vi "getBorderNum.vi"(0 "Refnum in":T1, 2 "Cut Limit":dbl format="%#_13g", 5 "Bounding Box":cluster{"x":sgl, "y":sgl}[][](array[cluster]), 7 "Position":sgl[][](array[numeric]), 9 "Angle":sgl[](array[numeric]), 11 "error in (no error)":errorcluster, 12 "Step":sgl=0.29742944, 13 "Origin Pixel":dbl[](array[numeric])) -> (4 "Refnum out":T1, 8 "Data Pieces":T3(array[cluster]) {"ROI Números"."Contours"."Type" items=["No Selection", "Point", "Line", "Rectangle", "Oval", "Polygon", "Freehand Region", "Annulus", "Unused2", "Unused3", "Broken Line", "Freehand Line", "Rotated Rectangle"]}, 15 "error out":errorcluster)   [LabVIEW 2016]
uses:
  <vilib>/vision/Image Controls.llb/IMAQ Image.ctl
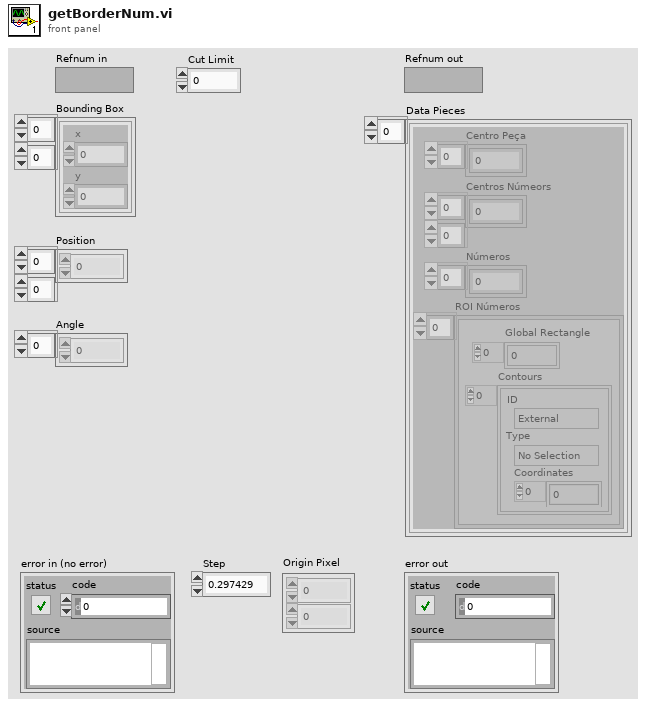
[diagram p1: front panel]
types:
  T1 = typedef "IMAQ Image.ctl" = refnum<image>
  T2 = typedef "ROI Descriptor" = cluster{"Global Rectangle":i32[], "Contours":cluster{"ID":enum32{"External", "Internal"}, "Type":u32, "Coordinates":i32[]}[]}
  T3 = cluster{"Centro Peça":dbl[], "Centros Númeors":dbl[][], "Números":u8[], "ROI Números":T2[]}[]
  T4 = cluster{"Centro Peça":dbl[], "Centros Númeors":dbl[][], "Números":u8[], "ROI Números":T2[]}
  T5 = typedef "IMAQ Rectangle" = cluster{"Left":i32, "Top":i32, "Right":i32, "Bottom":i32, "Rotation":dbl}
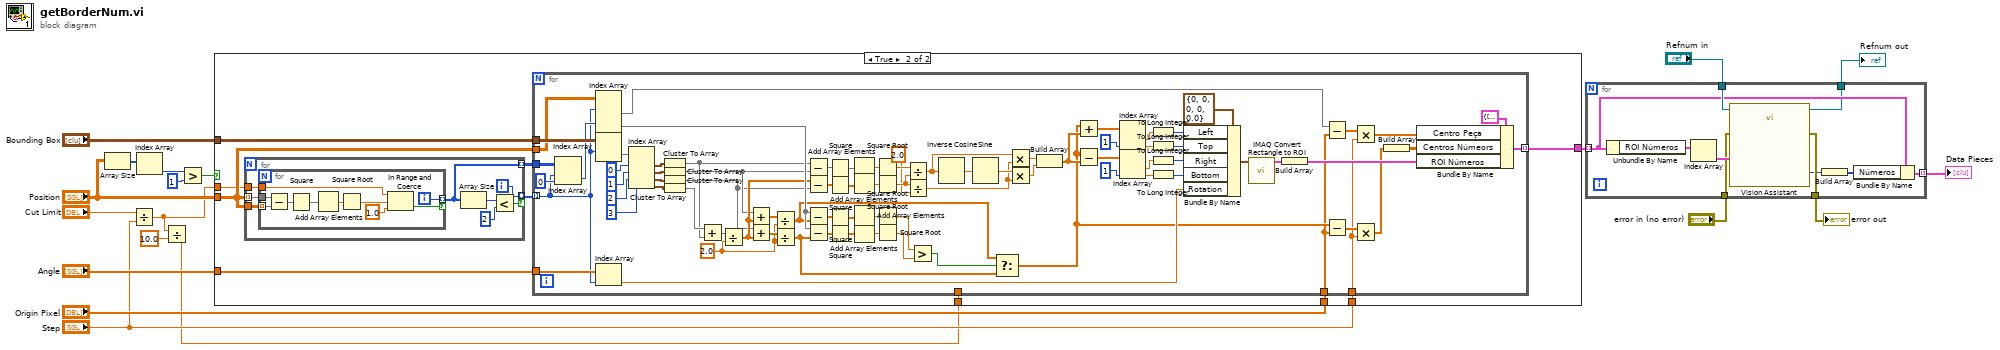
[diagram p0: block diagram]
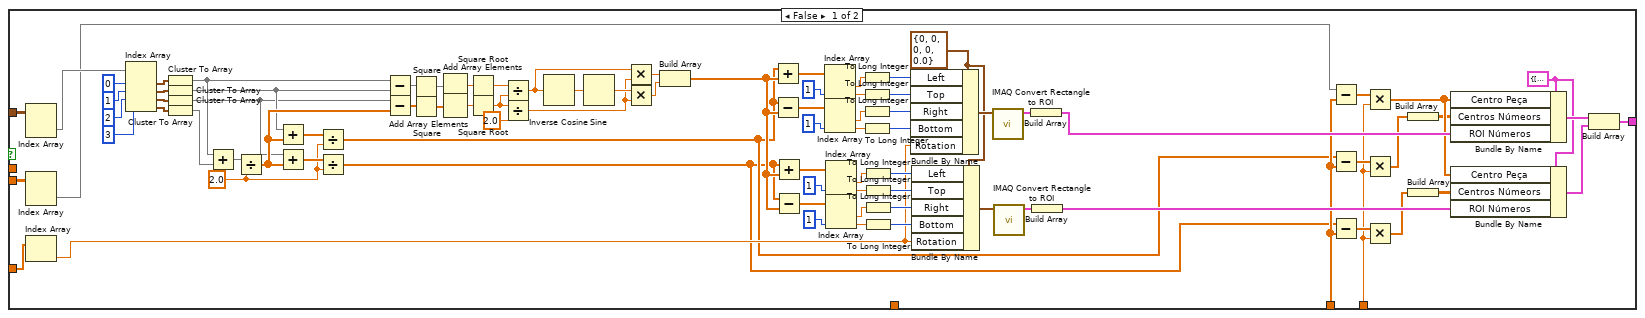
[diagram p2: hidden frame]
diagram:
  n1 = Array Size(array="Position") -> (size(s)=w9:i32[])
  n2 = Divide(x="Cut Limit", y="Step") -> (x/y=w3:dbl)
  n3 = Index Array(array=w9) -> (element=w10:i32)  [unwired: 1 in]
  n4 = Divide(x=w3, y=10.0) -> (x/y=w1:dbl)
  n5 = Greater?(x=w10, y=1) -> (0:w8:bool)
  n6 = case shown="True" w8 {
    tunnel: "Bounding Box" -> [w105 w115]
    tunnel: "Position" -> [w104 w114]
    tunnel: "Angle" -> [w43 w112]
    tunnel: [w39 w110] -> w14
    tunnel: w3 -> [_ w109]
    tunnel: "Origin Pixel" -> [w26 w108]
    tunnel: "Step" -> [w27 w107]
    tunnel: w1 -> [_ w106]
    frame False {
      w38 = T4 {"Centro Peça"=[0.0, 0.0], "Centros Númeors"=[[0.0, 0.0], [0.0, 0.0]], "Números"=[0, 0], "ROI Números"=[]} ("Dados Peça")
      w44 = T5 {"Left"=0, "Top"=0, "Right"=0, "Bottom"=0, "Rotation"=0.0} ("Rectangle")
      w80 = 2.0 ("y")
      n7 = Index Array(array=w105) -> (element=w103:cluster{"x":sgl, "y":sgl}[])  [unwired: 2 in]
      n8 = Index Array(array=w104) -> (element=w31:sgl[])  [unwired: 2 in]
      n9 = Index Array(array=w43) -> (element=w42:sgl)  [unwired: 1 in]
      n10 = Index Array(array=w103, index #1=0 ("index"), index #2=1 ("index"), index #3=2 ("index"), index #4=3 ("index")) -> (element #1=w98:cluster{"x":sgl, "y":sgl}, element #2=w97:cluster{"x":sgl, "y":sgl}, element #3=w96:cluster{"x":sgl, "y":sgl}, element #4=w95:cluster{"x":sgl, "y":sgl})
      n11 = Cluster To Array(cluster=w98) -> (array=w86:sgl[])
      n12 = Cluster To Array(cluster=w97) -> (array=w84:sgl[])
      n13 = Cluster To Array(cluster=w96) -> (array=w83:sgl[])
      n14 = Cluster To Array(cluster=w95) -> (array=w91:sgl[])
      n15 = Add(x=w86, y=w91) -> (x+y=w90:sgl[])
      n16 = Divide(x=w90, y=w80) -> (x/y=w85:dbl[])
      n17 = Add(x=w84, y=w85) -> (x+y=w82:dbl[])
      n18 = Add(x=w83, y=w85) -> (x+y=w81:dbl[])
      n19 = Divide(x=w82, y=w80) -> (x/y=w25:dbl[])
      n20 = Divide(x=w81, y=w80) -> (x/y=w24:dbl[])
      n21 = Subtract(x=w86, y=w84) -> (x-y=w87:sgl[])
      n22 = Subtract(x=w83, y=w85) -> (x-y=w92:dbl[])
      n23 = Square(x=w87) -> (x^2=w89:sgl[])
      n24 = Square(x=w92) -> (x^2=w94:dbl[])
      n25 = Add Array Elements(numeric array=w89) -> (sum=w88:sgl)
      n26 = Add Array Elements(numeric array=w94) -> (sum=w93:dbl)
      n27 = Square Root(x=w88) -> (sqrt(x)=w79:sgl)
      n28 = Square Root(x=w93) -> (sqrt(x)=w78:dbl)
      n29 = Divide(x=w79, y=w78) -> (x/y=w72:dbl)
      n30 = Divide(x=w78, y=2.0) -> (x/y=w71:dbl)
      n31 = Inverse Cosine(1:w72) -> (0:w76:dbl)
      n32 = Sine(x=w76) -> (sin(x)=w75:dbl)
      n33 = Multiply(x=w72, y=w71) -> (x*y=w73:dbl)
      n34 = Multiply(x=w75, y=w71) -> (x*y=w74:dbl)
      n35 = Build Array(w73, w74) -> (w41:dbl[])
      n36 = Add(x=w25, y=w41) -> (x+y=w58:dbl[])
      n37 = Subtract(x=w25, y=w41) -> (x-y=w59:dbl[])
      n38 = Add(x=w24, y=w41) -> (x+y=w45:dbl[])
      n39 = Subtract(x=w24, y=w41) -> (x-y=w46:dbl[])
      n40 = Index Array(array=w58, index #2=1 ("index")) -> (element #1=w60:dbl, element #2=w61:dbl)  [unwired: 1 in]
      n41 = Index Array(array=w59, index #2=1 ("index")) -> (element #1=w62:dbl, element #2=w63:dbl)  [unwired: 1 in]
      n42 = Index Array(array=w45, index #2=1 ("index")) -> (element #1=w47:dbl, element #2=w48:dbl)  [unwired: 1 in]
      n43 = Index Array(array=w46, index #2=1 ("index")) -> (element #1=w49:dbl, element #2=w50:dbl)  [unwired: 1 in]
      n44 = To Long Integer(number=w60) -> (32bit integer=w67:i32)
      n45 = To Long Integer(number=w61) -> (32bit integer=w66:i32)
      n46 = To Long Integer(number=w62) -> (32bit integer=w65:i32)
      n47 = To Long Integer(number=w63) -> (32bit integer=w64:i32)
      n48 = To Long Integer(number=w47) -> (32bit integer=w54:i32)
      n49 = To Long Integer(number=w48) -> (32bit integer=w53:i32)
      n50 = To Long Integer(number=w49) -> (32bit integer=w52:i32)
      n51 = To Long Integer(number=w50) -> (32bit integer=w51:i32)
      n52 = Bundle By Name(cluster=w44, "Left"=w67, "Top"=w66, "Right"=w65, "Bottom"=w64, "Rotation"=w42) -> (w68:T5)
      n53 = Bundle By Name(cluster=w44, "Left"=w54, "Top"=w53, "Right"=w52, "Bottom"=w51, "Rotation"=w42) -> (w55:T5)
      n54 = call "IMAQ Convert Rectangle to ROI"("Rectangle"=w68) -> ("ROI Descriptor"=w37:T2)  [unwired: 8 in, 1 out]
      n55 = call "IMAQ Convert Rectangle to ROI"("Rectangle"=w55) -> ("ROI Descriptor"=w36:T2)  [unwired: 8 in, 1 out]
      n56 = Build Array(w37) -> (w34:T2[])
      n57 = Build Array(w36) -> (w35:T2[])
      n58 = Subtract(x=w31, y=w26) -> (x-y=w32:dbl[])
      n59 = Subtract(x=w25, y=w26) -> (x-y=w29:dbl[])
      n60 = Subtract(x=w24, y=w26) -> (x-y=w28:dbl[])
      n61 = Multiply(x=w32, y=w27) -> (x*y=w30:dbl[])
      n62 = Multiply(x=w29, y=w27) -> (x*y=w23:dbl[])
      n63 = Multiply(x=w28, y=w27) -> (x*y=w20:dbl[])
      n64 = Build Array(w23) -> (w22:dbl[][])
      n65 = Build Array(w20) -> (w21:dbl[][])
      n66 = Bundle By Name(cluster=w38, "Centro Peça"=w30, "Centros Númeors"=w22, "ROI Números"=w34) -> (w40:T4)
      n67 = Bundle By Name(cluster=w38, "Centro Peça"=w30, "Centros Númeors"=w21, "ROI Números"=w35) -> (w33:T4)
      n68 = Build Array(w40, w33) -> (w39:T3)
    }
    frame True {
      n69 = for {
        tunnel: w114 -> [w204] mode=indexing
        tunnel: w114 -> [w203]
        tunnel: [w202] -> w113 mode=indexing if=w199
        tunnel: [w198] -> w111 mode=indexing
        tunnel: w109 -> [w197]
        i -> [w202]
        n70 = for {
          tunnel: w204 -> [w214]
          tunnel: w203 -> [w210] mode=indexing
          tunnel: [w207] -> w198 mode=indexing if=w206
          tunnel: w197 -> [w205]
          i -> [w207]
          n71 = Subtract(x=w214, y=w210) -> (x-y=w213:sgl[])
          n72 = Square(x=w213) -> (x^2=w212:sgl[])
          n73 = Add Array Elements(numeric array=w212) -> (sum=w211:sgl)
          n74 = Square Root(x=w211) -> (sqrt(x)=w208:sgl)
          n75 = In Range and Coerce(upper limit=w205, x=w208, lower limit=1.0) -> (In Range?=w206:bool)  [unwired: 1 out]
        }
        n76 = Array Size(array=w198) -> (size(s)=w201:i32)
        n77 = Less?(x=w201, y=2) -> (x < y?=w199:bool)
      }
      n78 = for {
        tunnel: w115 -> [w196]
        tunnel: w114 -> [w194]
        tunnel: w113 -> [w156] mode=indexing
        tunnel: w112 -> [w182]
        tunnel: w111 -> [w179]
        tunnel: [w128] -> w110 mode=indexing
        tunnel: w108 -> [w120]
        tunnel: w107 -> [w119]
        tunnel: w106 -> [_]
        w155 = 2.0 ("y")
        n79 = Index Array(array=w179, index (row)=w156, index (col)=0 ("disabled index (col)")) -> (element=w178:i32)
        n80 = Index Array(array=w194, index (row) #1=w156, index (row) #2=w178) -> (element #1=w127:sgl[], element #2=w157:sgl[])  [unwired: 2 in]
        n81 = Index Array(array=w196, index (row)=w156) -> (element=w195:cluster{"x":sgl, "y":sgl}[])  [unwired: 1 in]
        n82 = Index Array(array=w182, index=w156) -> (element=w181:sgl)
        n83 = Index Array(array=w195, index #1=0 ("index"), index #2=1 ("index"), index #3=2 ("index"), index #4=3 ("index")) -> (element #1=w192:cluster{"x":sgl, "y":sgl}, element #2=w193:cluster{"x":sgl, "y":sgl}, element #3=w191:cluster{"x":sgl, "y":sgl}, element #4=w174:cluster{"x":sgl, "y":sgl})
        n84 = Cluster To Array(cluster=w192) -> (array=w144:sgl[])
        n85 = Cluster To Array(cluster=w193) -> (array=w143:sgl[])
        n86 = Cluster To Array(cluster=w191) -> (array=w138:sgl[])
        n87 = Cluster To Array(cluster=w174) -> (array=w171:sgl[])
        n88 = Add(x=w171, y=w144) -> (x+y=w173:sgl[])
        n89 = Divide(x=w173, y=w155) -> (x/y=w149:dbl[])
        n90 = Add(x=w143, y=w149) -> (x+y=w148:dbl[])
        n91 = Add(x=w138, y=w149) -> (x+y=w170:dbl[])
        n92 = Divide(x=w148, y=w155) -> (x/y=w154:dbl[])
        n93 = Divide(x=w170, y=w155) -> (x/y=w153:dbl[])
        n94 = Subtract(x=w144, y=w143) -> (x-y=w145:sgl[])
        n95 = Subtract(x=w149, y=w138) -> (x-y=w152:dbl[])
        n96 = Subtract(x=w157, y=w154) -> (x-y=w169:dbl[])
        n97 = Subtract(x=w157, y=w153) -> (x-y=w158:dbl[])
        n98 = Square(x=w145) -> (x^2=w147:sgl[])
        n99 = Square(x=w152) -> (x^2=w150:dbl[])
        n100 = Square(x=w169) -> (x^2=w167:dbl[])
        n101 = Square(x=w158) -> (x^2=w160:dbl[])
        n102 = Add Array Elements(numeric array=w147) -> (sum=w146:sgl)
        n103 = Add Array Elements(numeric array=w150) -> (sum=w151:dbl)
        n104 = Add Array Elements(numeric array=w167) -> (sum=w168:dbl)
        n105 = Add Array Elements(numeric array=w160) -> (sum=w159:dbl)
        n106 = Square Root(x=w146) -> (sqrt(x)=w142:sgl)
        n107 = Square Root(x=w151) -> (sqrt(x)=w137:dbl)
        n108 = Square Root(x=w168) -> (sqrt(x)=w118:dbl)
        n109 = Square Root(x=w159) -> (sqrt(x)=w117:dbl)
        n110 = Divide(x=w142, y=w137) -> (x/y=w139:dbl)
        n111 = Divide(x=w137, y=2.0) -> (x/y=w135:dbl)
        n112 = Greater?(x=w118, y=w117) -> (0:w116:bool)
        n113 = Inverse Cosine(1:w139) -> (0:w141:dbl)
        n114 = Sine(x=w141) -> (sin(x)=w140:dbl)
        n115 = Select(t=w154, s=w116, f=w153) -> (s? t:f=w121:dbl[])
        n116 = Multiply(x=w139, y=w135) -> (x*y=w133:dbl)
        n117 = Multiply(x=w140, y=w135) -> (x*y=w134:dbl)
        n118 = Build Array(w133, w134) -> (w132:dbl[])
        n119 = Add(x=w121, y=w132) -> (x+y=w161:dbl[])
        n120 = Subtract(x=w121, y=w132) -> (x-y=w162:dbl[])
        n121 = Index Array(array=w161, index #2=1 ("index")) -> (element #1=w163:dbl, element #2=w164:dbl)  [unwired: 1 in]
        n122 = Index Array(array=w162, index #2=1 ("index")) -> (element #1=w165:dbl, element #2=w166:dbl)  [unwired: 1 in]
        n123 = To Long Integer(number=w163) -> (32bit integer=w186:i32)
        n124 = To Long Integer(number=w164) -> (32bit integer=w185:i32)
        n125 = To Long Integer(number=w165) -> (32bit integer=w184:i32)
        n126 = To Long Integer(number=w166) -> (32bit integer=w183:i32)
        n127 = Bundle By Name(cluster=T5 {"Left"=0, "Top"=0, "Right"=0, "Bottom"=0, "Rotation"=0.0} ("Rectangle"), "Left"=w186, "Top"=w185, "Right"=w184, "Bottom"=w183, "Rotation"=w181) -> (w187:T5)
        n128 = call "IMAQ Convert Rectangle to ROI"("Rectangle"=w187) -> ("ROI Descriptor"=w130:T2)  [unwired: 8 in, 1 out]
        n129 = Build Array(w130) -> (w129:T2[])
        n130 = Subtract(x=w127, y=w120) -> (x-y=w126:dbl[])
        n131 = Subtract(x=w121, y=w120) -> (x-y=w124:dbl[])
        n132 = Multiply(x=w126, y=w119) -> (x*y=w125:dbl[])
        n133 = Multiply(x=w124, y=w119) -> (x*y=w122:dbl[])
        n134 = Build Array(w122) -> (w123:dbl[][])
        n135 = Bundle By Name(cluster=T4 {"Centro Peça"=[0.0, 0.0], "Centros Númeors"=[[0.0, 0.0], [0.0, 0.0]], "Números"=[0, 0], "ROI Números"=[]} ("Dados Peça"), "Centro Peça"=w125, "Centros Númeors"=w123, "ROI Números"=w129) -> (w128:T4)
      }
    }
  }
  n136 = for {
    tunnel: w14 -> [w220] mode=indexing
    tunnel: "Refnum in" -> [w222]
    tunnel: [w221] -> w15
    tunnel: [w217] -> w16 mode=indexing
    tunnel: "error in (no error)" -> [w216]
    tunnel: [w215] -> w7
    n137 = Unbundle By Name(w220) -> ("ROI Números"=w224:T2[])
    n138 = Index Array(array=w224) -> (element=w223:T2)  [unwired: 1 in]
    n139 = call "Vision Assistant"("Image In"=w222, "ROI Descriptor (Image Mask 1)"=w223, "error in"=w216) -> ("Image Out"=w215:T1, "Number of Particles (Particle Analysis 1)"=w219:i32, "error out"=w221:errorcluster)  [unwired: 22 in]
    n140 = Build Array(w219) -> (w218:i32[])
    n141 = Bundle By Name(cluster=w220, "Números"=w218) -> (w217:T4)
  }
  "Data Pieces" <- w16
  "error out" <- w15
  "Refnum out" <- w7
